vi "SetComment.vi"(8 "error in (no error)":errorcluster, 11 "ActionEditor in":refnum<class "ActionEditor.lvclass">) -> (0 "error out":errorcluster, 3 "ActionEditor out":refnum<class "ActionEditor.lvclass">)   [LabVIEW 2011, in "Views.lvlib" / "ScriptEditor.lvlib" / "ActionEditor.lvclass"]
uses:
  ActionEditor.lvclass
  ActionEditor.lvclass/ActionEditor.ctl
  Tools/Scripting/ScriptingEvent/ScriptEvent.lvclass
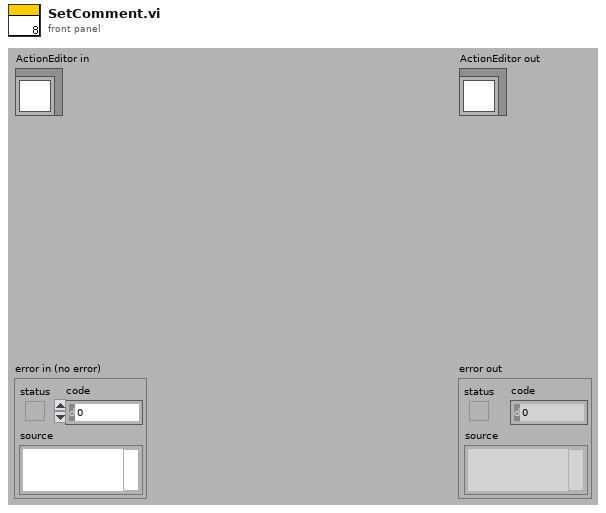
[diagram p1: front panel]
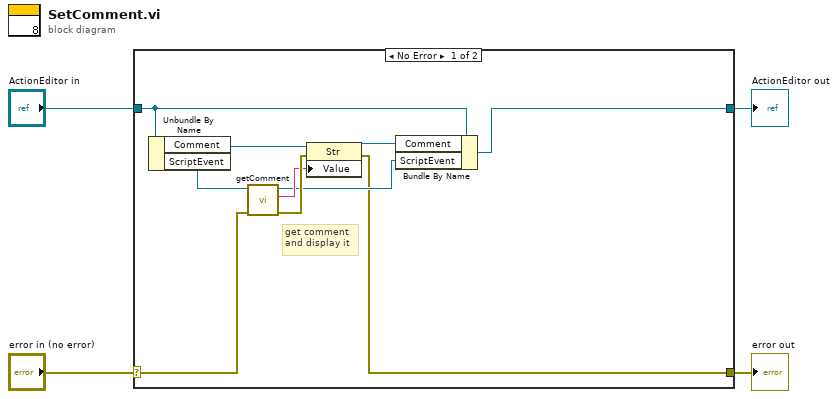
[diagram p0: block diagram]
diagram:
  n1 = case shown="No Error" "error in (no error)" {
    selector: "error in (no error)" -> [w13 w16]
    tunnel: [w5 w16] -> w3
    tunnel: [w6 w15] -> w1
    tunnel: "ActionEditor in" -> [w7 w15]
    frame No Error {
      # "get comment\nand display it"
      n2 = Unbundle By Name(w7) -> ("Comment"=w12:refnum<vi>, "ScriptEvent"=w14:refnum<class "ScriptEvent.lvclass">)
      n3 = call "getComment.vi"("error in (no error)"=w13, "ScriptEvent.lvclass in"=w14) -> ("error out"=w11:errorcluster, "comment"=w10:string, "ScriptEvent.lvclass out"=w8:refnum<class "ScriptEvent.lvclass">)  [unwired: 7 in]
      n4 = property class="Str"(reference=w12, error in=w11, "Value"=w10) -> (reference out=w9:refnum<vi>, error out=w5:errorcluster)
      n5 = Bundle By Name(cluster=w7, "Comment"=w9, "ScriptEvent"=w8) -> (w6:refnum<class "ActionEditor.lvclass">)
    }
    frame Error {
    }
  }
  "error out" <- w3
  "ActionEditor out" <- w1
